vi "testing odor-manifold-stim config v2.vi"() -> ()   [LabVIEW 2021]
uses:
  type-defs/stimulation configuration array (type def).ctl
  type-defs/stimulator configuration line cluster (type def).ctl
  type-defs/port-odor with color cluster (type def).ctl
  type-defs/port-odor ring (type def).ctl
  type-defs/odor color (type def).ctl
  type-defs/odor and manifold config cluster (type def).ctl
  type-defs/manifold configuration cluster array (type def).ctl
  type-defs/manifold configuration cluster (type def).ctl
  type-defs/manifold selection.ctl
  type-defs/single port single odor cluster.ctl
  type-defs/port number (type def).ctl
  type-defs/odor selection (type def).ctl
  type-defs/odor description array (type def).ctl
  type-defs/odor info cluster (type def).ctl
  type-defs/ragged ring entry 2D array cluster (typed def).ctl
  type-defs/ring string and value cluster (type def).ctl
  type-defs/stimulation config UI states (type def).ctl
  <vilib>/ErrorRing/Error Ring.xnode
panel:
  out "changed rows":bool[](array[boolean])
  out "value error":errorcluster
  out "error out":errorcluster
  out "ragged ring entry 2D array":T1
  out "odor & manifold config cluster":T3
  out "odor-manifold config ok?":bool
  in  "stim. config array":T13 {"right odor"."port-odor ring" items=["off"=0, "fish water, 3 <Odor:3, Port:0>"=3, "alarm substance <Odor:5, Port:1>"=5]; "middle odor"."port-odor ring" items=["off"=0, "fish water, 2 <Odor:2, Port:0>"=2]; "left odor"."port-odor ring" items=["off"=0, "fish water, 1 <Odor:1, Port:0>"=1, "alanine <Odor:4, Port:1>"=4]; "duration, s" format="%.1f"}
  in  "Stop":bool
  in  "configure odor-manifold":bool
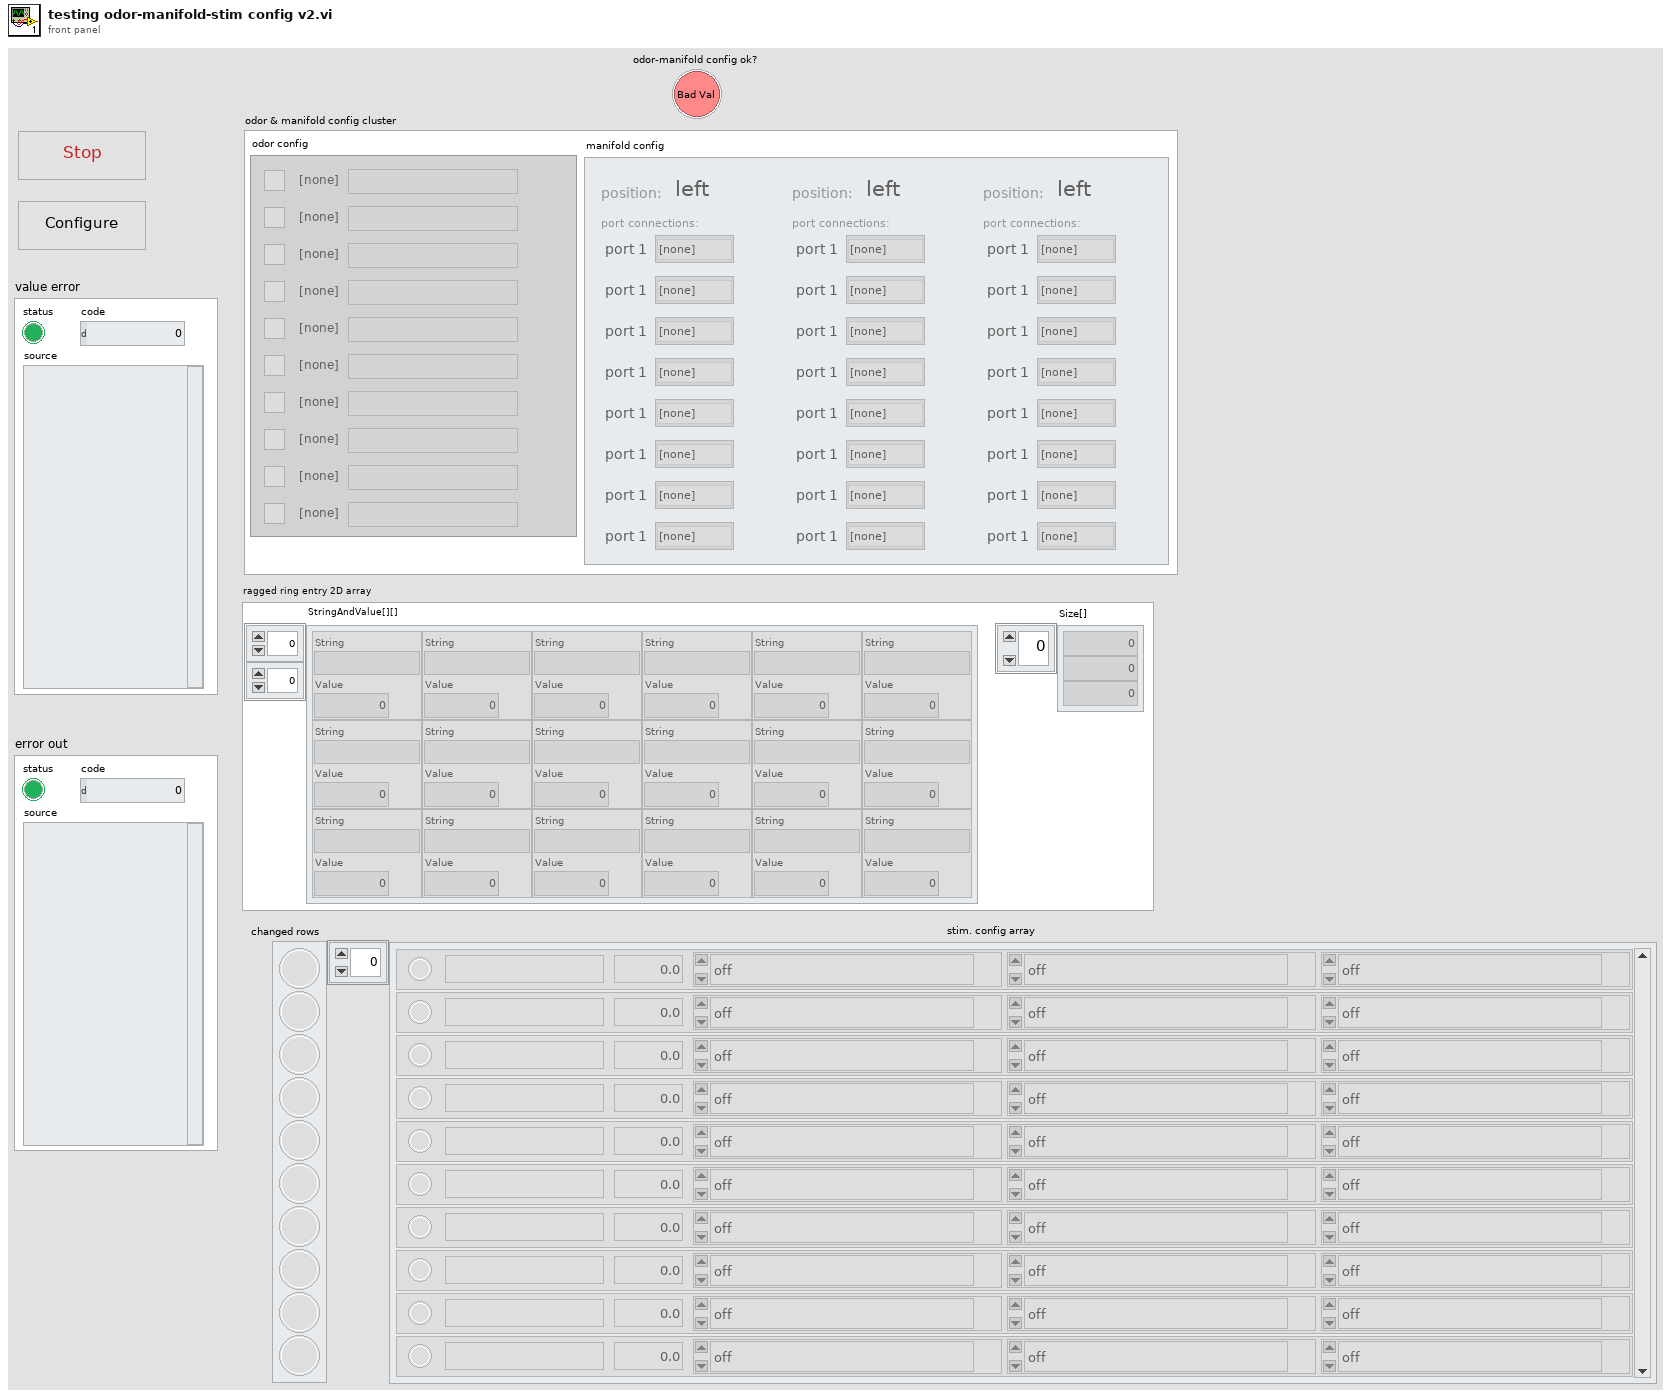
[diagram p1: front panel]
types:
  T1 = typedef "ragged ring entry 2D array cluster (typed def).ctl" = cluster{"StringAndValue[][]":T2[][], "Size[]":i32[]}
  T2 = typedef "ring string and value cluster (type def).ctl" = cluster{"String":string, "Value":u16}
  T3 = typedef "odor and manifold config cluster (type def).ctl" = cluster{"manifold config":T4, "odor config":T11}
  T4 = typedef "manifold configuration cluster array (type def).ctl" = T5[]
  T5 = typedef "manifold configuration cluster (type def).ctl" = cluster{"position:":T6, "port connections:":T7[]}
  T6 = typedef "manifold selection.ctl" = enum16{"left", "middle", "right"}
  T7 = typedef "single port single odor cluster.ctl" = cluster{"port number":T8, "connected odor":T9, "error":bool, "odor color":T10}
  T8 = typedef "port number (type def).ctl" = enum16{"port 1", "port 2", "port 3", "port 4", "port 5", "port 6", "port 7", "port 8"}
  T9 = typedef "odor selection (type def).ctl" = enum16{"[none]", "odor 1", "odor 2", "odor 3", "odor 4", "odor 5", "odor 6", "odor 7", "odor 8", "odor 9", "odor 10"}
  T10 = typedef "odor color (type def).ctl" = u16
  T11 = typedef "odor description array (type def).ctl" = T12[]
  T12 = typedef "odor info cluster (type def).ctl" = cluster{"odor channel":T9, "odor description":string, "odor color":T10, "odor channel active":bool}
  T13 = typedef "stimulation configuration array (type def).ctl" = T14[]
  T14 = typedef "stimulator configuration line cluster (type def).ctl" = cluster{"description":string, "duration, s":dbl, "left odor":T15, "middle odor":T15, "right odor":T15, "selected?":bool}
  T15 = typedef "port-odor with color cluster (type def).ctl" = cluster{"port-odor ring":T16, "odor color":T10}
  T16 = typedef "port-odor ring (type def).ctl" = u16
  T17 = typedef "stimulation config UI states (type def).ctl" = enum16{"Initialize", "Wait For Event", "Open Odor-Manifold Dialog", "Update Stim Config", "Handle Errors", "Save Config to File", "Load Config from File", "Exit", "Crash"}
  T18 = enum8{"Enabled", "Disabled", "Disabled and Grayed Out"}
  T19 = cluster{"stim. config line cluster":refnum<vi>, "description string":refnum<vi>, "duration, s numeric":refnum<vi>, "port-odor & color cluster []":refnum<vi>[], "port-odor ring []":refnum<vi>[], "odor color ring []":refnum<vi>[]}
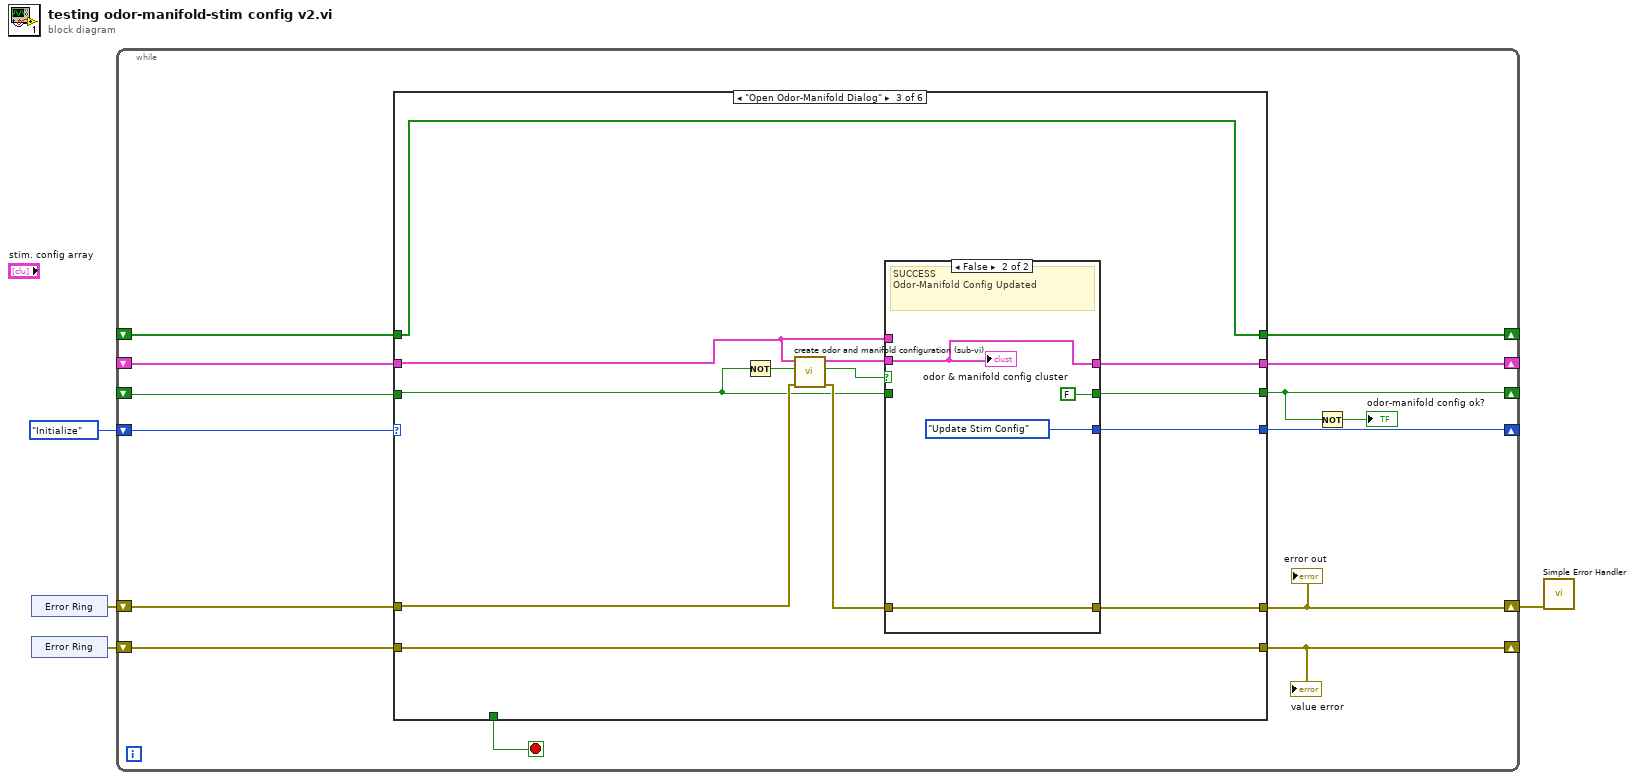
[diagram p0: block diagram]
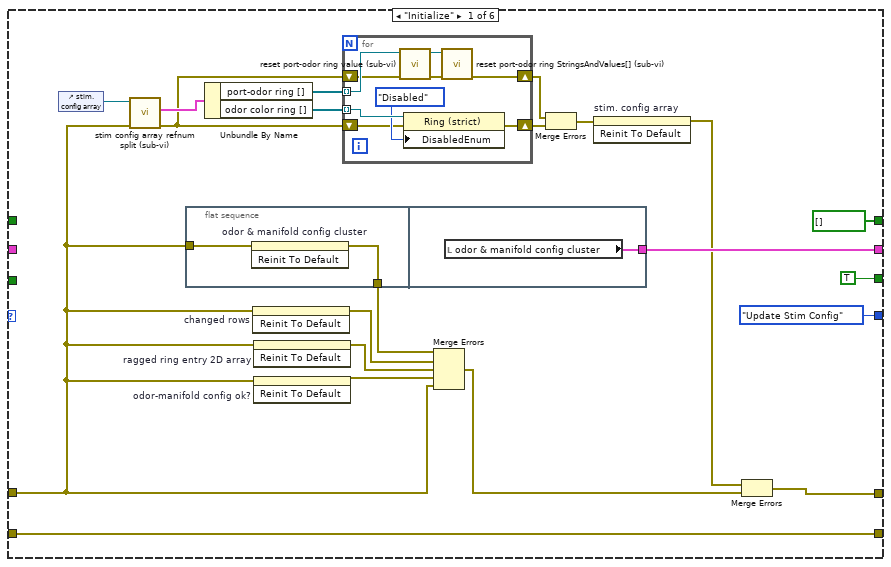
[diagram p2: hidden frame]
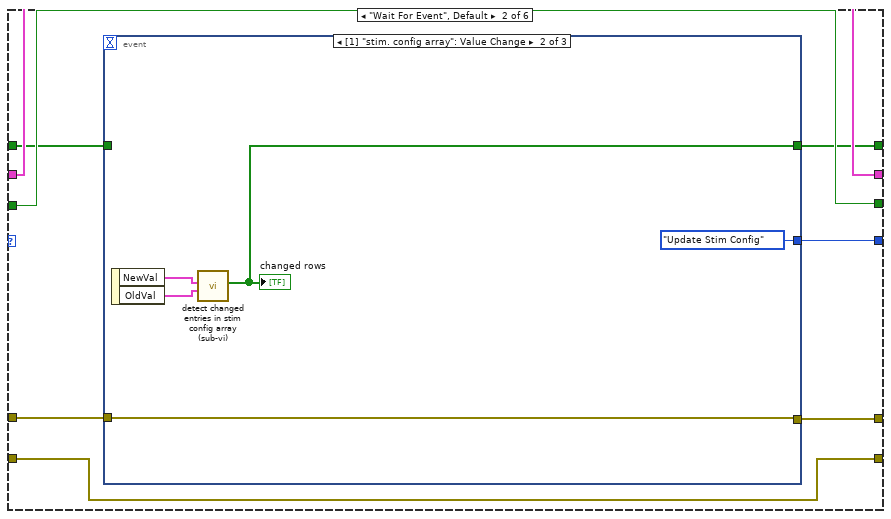
[diagram p3: hidden frame]
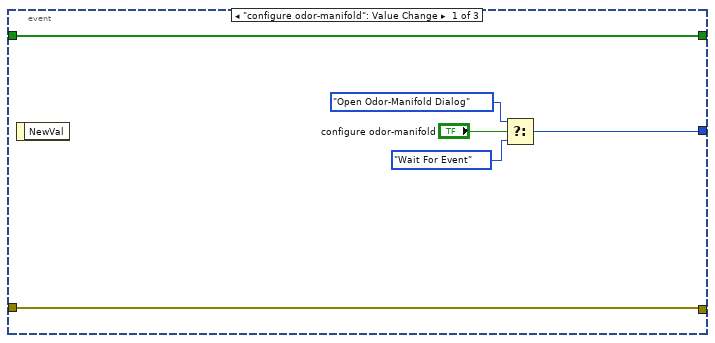
[diagram p4: hidden frame]
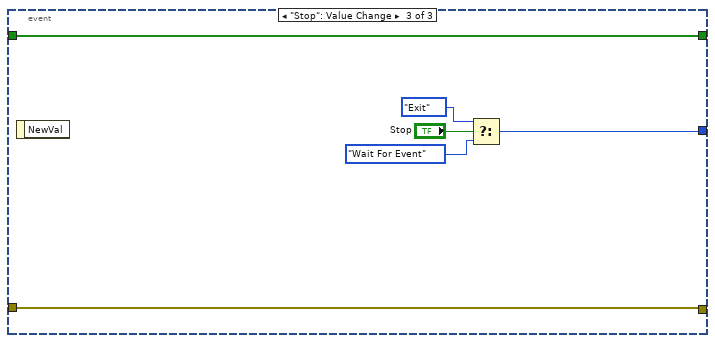
[diagram p5: hidden frame]
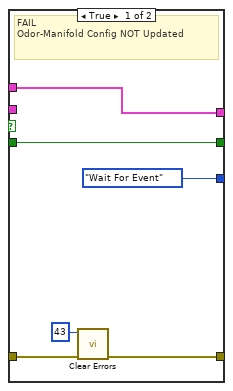
[diagram p6: hidden frame]
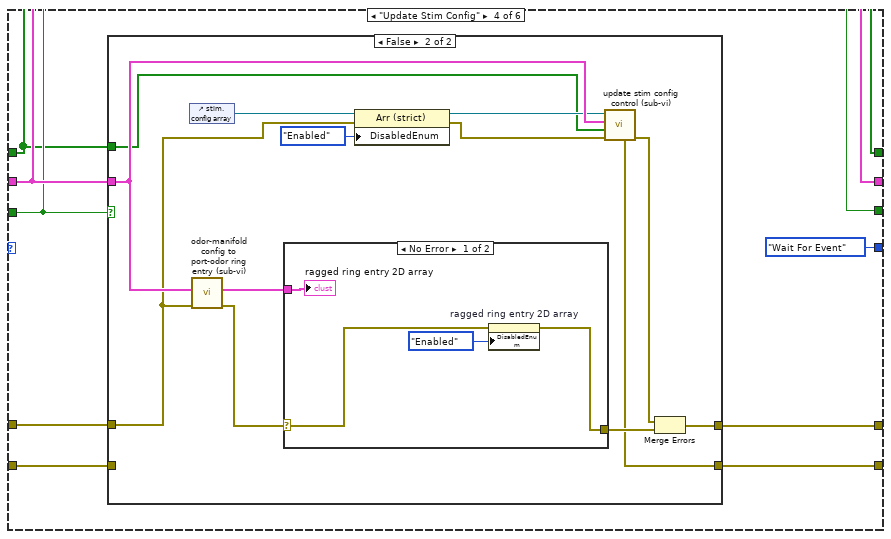
[diagram p7: hidden frame]
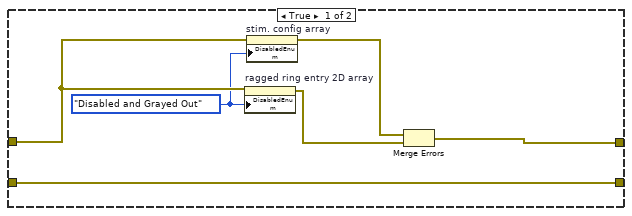
[diagram p8: hidden frame]
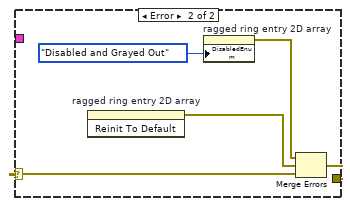
[diagram p9: hidden frame]
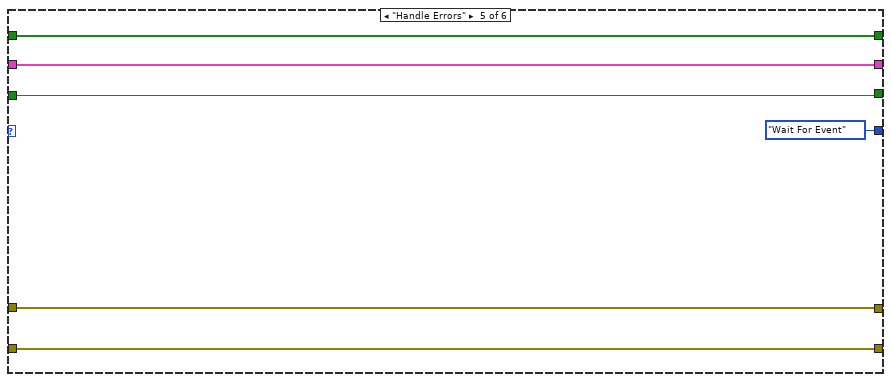
[diagram p10: hidden frame]
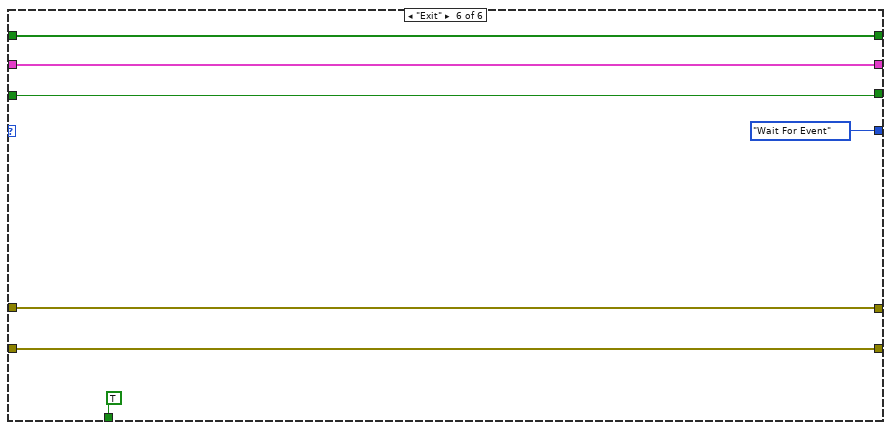
[diagram p11: hidden frame]
diagram:
  n1 = xnode "Error Ring"() -> ("error out"=w3:errorcluster)
  n2 = xnode "Error Ring"() -> ("error out"=w1:errorcluster)
  n3 = while {
    shift-right: [w8] -> _
    shift-left: _ -> [w18]
    shift-right: [w15] -> w2
    shift-left: w3 -> [w16]
    shift-right: [w13] -> _
    shift-left: stimulation_config_UI_states_(type_def)."Initialize" ("Enum") -> [w14]
    shift-right: [w12] -> _
    shift-left: _ -> [w11]
    shift-right: [w10] -> _
    shift-left: w1 -> [w9]
    shift-right: [w6] -> _
    shift-left: _ -> [w5]
    stop <- w17 stop-if-true
    n4 = case shown="\"Open Odor-Manifold Dialog\"" w14 {
      tunnel: w18 -> [_ w56 w82 w103 w141 w146]
      tunnel: [TRUE w56 w83 w103 w141 w146] -> w8
      tunnel: [_ _ _ _ _ TRUE ("NewVal")] -> w17
      tunnel: w16 -> [w24 w59 w85 w106 w139 w147]
      tunnel: [w34 w58 w84 w105 w139 w147] -> w15
      tunnel: [stimulation_config_UI_states_(type_def)."Update Stim Config" ("Enum") w57 w81 stimulation_config_UI_states_(type_def)."Wait For Event" ("Enum") stimulation_config_UI_states_(type_def)."Wait For Event" ("Enum") stimulation_config_UI_states_(type_def)."Wait For Event" ("Enum")] -> w13
      tunnel: [w30 w55 w80 w104 w138 w144] -> w12
      tunnel: w11 -> [_ w55 w79 w104 w138 w144]
      tunnel: [w33 w54 w78 w102 w137 w143] -> w10
      tunnel: w9 -> [w33 w54 w78 w101 w137 w143]
      tunnel: [bool[] [] ("[ changed? ]") w53 w77 w100 w136 w142] -> w6
      tunnel: w5 -> [_ w52 w77 w100 w136 w142]
      frame "Initialize" {
        n5 = control-ref of="stim. config array"() -> (w37:refnum<vi>)
        n6 = call "stim config array refnum split (sub-vi).vi"("error in (no error)"=w24, "stim. config array refnum"=w37) -> ("error out"=w25:errorcluster, "element refnum cluster"=w36:T19)  [unwired: 7 in, 1 out]
        n7 = flat-sequence {
          tunnel: [w41] -> w28
          tunnel: w24 -> [w40]
          tunnel: [w42] -> w30
          frame #0 {
            n8 = invoke on="odor & manifold config cluster" class="Clust (strict)" method="Reinit To Default"(error in=w40) -> (error out=w41:errorcluster)  [unwired: 2 in, 2 out]
          }
          frame #1 {
            n9 = local read "odor & manifold config cluster"() -> (w42:T3)
          }
        }
        n10 = Unbundle By Name(w36) -> ("port-odor ring []"=w26:refnum<vi>[], "odor color ring []"=w35:refnum<vi>[])
        n11 = invoke on="changed rows" class="Arr (strict)" method="Reinit To Default"(error in=w24) -> (error out=w27:errorcluster)  [unwired: 2 in, 2 out]
        n12 = invoke on="ragged ring entry 2D array" class="Clust (strict)" method="Reinit To Default"(error in=w24) -> (error out=w31:errorcluster)  [unwired: 2 in, 2 out]
        n13 = invoke on="odor-manifold config ok?" class="Bool (strict)" method="Reinit To Default"(error in=w24) -> (error out=w32:errorcluster)  [unwired: 2 in, 2 out]
        n14 = for {
          tunnel: w35 -> [w51] mode=indexing
          shift-right: [w48] -> w22
          shift-left: w25 -> [w49]
          tunnel: w26 -> [w45] mode=indexing
          shift-right: [w43] -> w23
          shift-left: w25 -> [w44]
          n15 = call "reset port-odor ring value (sub-vi).vi"("error in (no error)"=w44, "port-odor ring refnum"=w45) -> ("error out"=w47:errorcluster, "port-odor ring refnum out"=w46:refnum<vi>)  [unwired: 8 in]
          n16 = property class="Ring (strict)"(reference=w51, error in=w49, "DisabledEnum"=T18."Disabled" ("Disabled")) -> (error out=w48:errorcluster)  [unwired: 1 out]
          n17 = call "reset port-odor ring StringsAndValues[] (sub-vi).vi"("error in (no error)"=w47, "port-odor ring refnum"=w46) -> ("error out"=w43:errorcluster)  [unwired: 8 in, 1 out]
        }
        n18 = Merge Errors(w28, w27, w31, w32, w24) -> (w38:errorcluster)
        n19 = Merge Errors(w23, w22) -> (w21:errorcluster)
        n20 = invoke on="stim. config array" class="Arr (strict)" method="Reinit To Default"(error in=w21) -> (error out=w20:errorcluster)  [unwired: 2 in, 2 out]
        n21 = Merge Errors(w20, w38) -> (w34:errorcluster)
      }
      frame "Wait For Event", Default {
        n22 = event shown="[1] \"stim. config array\": Value Change" {
          selector: _ -> [_ _ _]
          dyn-events: _ -> [_ _ _]
          timeout: _ -> [_ _ _]
          tunnel: w59 -> [w65 w69 w76]
          tunnel: [w65 w69 w76] -> w58
          tunnel: [w61 stimulation_config_UI_states_(type_def)."Update Stim Config" ("Enum") w72] -> w57
          tunnel: [w60 w66 w71] -> w53
          tunnel: w52 -> [w60 _ w71]
          event "configure odor-manifold": Value Change {
            n23 = event-data() -> ()  [unwired: 1 in, 1 out]
            n24 = Select(t=stimulation_config_UI_states_(type_def)."Open Odor-Manifold Dialog" ("Enum"), s="configure odor-manifold", f=stimulation_config_UI_states_(type_def)."Wait For Event") -> (s? t:f=w61:T17)
          }
          event Value Change {
            n25 = event-data() -> ("NewVal"=w68:T13, "OldVal"=w67:T13)  [unwired: 1 in]
            n26 = call "detect changed entries in stim config array (sub-vi).vi"("OLD stim. config array"=w67, "NEW stim. config array"=w68) -> ("[ changed? ]"=w66:bool[])  [unwired: 9 in]
            "changed rows" <- w66
          }
          event "Stop": Value Change {
            n27 = event-data() -> ()  [unwired: 1 in, 1 out]
            n28 = Select(t=stimulation_config_UI_states_(type_def)."Exit" ("Enum"), s="Stop", f=stimulation_config_UI_states_(type_def)."Wait For Event" ("Enum")) -> (s? t:f=w72:T17)
          }
        }
      }
      frame "Open Odor-Manifold Dialog" {
        n29 = Not(x=w82) -> (.not. x?=w87:bool)
        n30 = call "create odor and manifold configuration (sub-vi).vi"("error in (no error)"=w85, "use initial config? (F)"=w87, "initial odor and manifold config (none)"=w79) -> ("error out"=w86:errorcluster, "operation failed?"=w88:bool, "odor and manifold config out"=w89:T3)  [unwired: 6 in]
        n31 = case shown="False" w88 {
          tunnel: w89 -> [_ w96]
          tunnel: w82 -> [w95 _]
          tunnel: [w95 FALSE] -> w83
          tunnel: w86 -> [w94 w98]
          tunnel: [w93 w98] -> w84
          tunnel: [stimulation_config_UI_states_(type_def)."Wait For Event" ("Enum") stimulation_config_UI_states_(type_def)."Update Stim Config" ("Enum")] -> w81
          tunnel: [w90 w96] -> w80
          tunnel: w79 -> [w90 _]
          frame True {
            # "FAIL\nOdor-Manifold Config NOT Updated"
            n32 = call <vilib>:"Clear Errors.vi"("error in (no error)"=w94, "specific error code to clear (0: all)"=43) -> ("error out"=w93:errorcluster)  [unwired: 4 in, 1 out]
          }
          frame False {
            # "SUCCESS\nOdor-Manifold Config Updated"
            "odor & manifold config cluster" <- w96
          }
        }
      }
      frame "Update Stim Config" {
        n33 = case shown="False" w103 {
          tunnel: w106 -> [w111 w117]
          tunnel: [w109 w122] -> w105
          tunnel: w104 -> [_ w123]
          tunnel: [w112 w120] -> w102
          tunnel: w101 -> [w112 _]
          tunnel: w100 -> [_ w114]
          frame True {
            w110 = T18."Disabled and Grayed Out" ("Disabled")
            n34 = property on="ragged ring entry 2D array" class="Clust (strict)"(error in=w111, "DisabledEnum"=w110) -> (error out=w113:errorcluster)  [unwired: 1 in, 1 out]
            n35 = property on="stim. config array" class="Arr (strict)"(error in=w111, "DisabledEnum"=w110) -> (error out=w108:errorcluster)  [unwired: 1 in, 1 out]
            n36 = Merge Errors(w108, w113) -> (w109:errorcluster)
          }
          frame False {
            n37 = control-ref of="stim. config array"() -> (w119:refnum<vi>)
            n38 = call "odor-manifold config to port-odor ring entry (sub-vi).vi"("error in (no error)"=w117, "odor-manifold config"=w123) -> ("error out"=w125:errorcluster, "ragged ring entry 2D array"=w126:T1)  [unwired: 8 in]
            n39 = case shown="No Error" w125 {
              selector: w125 -> [w128 w131]
              tunnel: w126 -> [w130 _]
              tunnel: [w127 w132] -> w124
              frame No Error {
                n40 = property on="ragged ring entry 2D array" class="Clust (strict)"(error in=w128, "DisabledEnum"=T18."Enabled" ("Disabled")) -> (error out=w127:errorcluster)  [unwired: 1 in, 1 out]
                "ragged ring entry 2D array" <- w130
              }
              frame Error {
                n41 = invoke on="ragged ring entry 2D array" class="Clust (strict)" method="Reinit To Default"() -> (error out=w133:errorcluster)  [unwired: 3 in, 2 out]
                n42 = property on="ragged ring entry 2D array" class="Clust (strict)"("DisabledEnum"=T18."Disabled and Grayed Out" ("Disabled")) -> (error out=w134:errorcluster)  [unwired: 2 in, 1 out]
                n43 = Merge Errors(w134, w133, w131) -> (w132:errorcluster)
              }
            }
            n44 = property class="Arr (strict)"(reference=w119, error in=w117, "DisabledEnum"=T18."Enabled" ("Disabled")) -> (reference out=w118:refnum<vi>, error out=w116:errorcluster)
            n45 = call "update stim config control (sub-vi).vi"("error in (no error)"=w116, "changed? [] (empty)"=w114, "odor-manifold config"=w123, "stim. config array refnum"=w118) -> ("error out"=w121:errorcluster, "value error"=w120:errorcluster)  [unwired: 5 in, 1 out]
            n46 = Merge Errors(w121, w124) -> (w122:errorcluster)
          }
        }
      }
      frame "Handle Errors" {
      }
      frame "Exit" {
      }
    }
    "error out" <- w15
    "value error" <- w10
    n47 = Not(x=w8) -> (.not. x?=→"odor-manifold config ok?":bool)
  }
  n48 = call <vilib>:"Simple Error Handler.vi"("error in (no error)"=w2) -> ()  [unwired: 4 in, 5 out]
